vi "runningseperately.vi"() -> ()   [LabVIEW 2019]
uses:
  <vilib>/Utility/file.llb/Read Delimited Spreadsheet (DBL).vi
panel:
  out "Torque Setpoints_graph":dbl(graph)
  in  "Tyre Diameter(m)":sgl=0.78
  in  "file path (dialog if empty)":path=path "C:/Users/arda/Documents/GitHub/labviewtestbench/RPM_setpointfile/wholetest.txt"
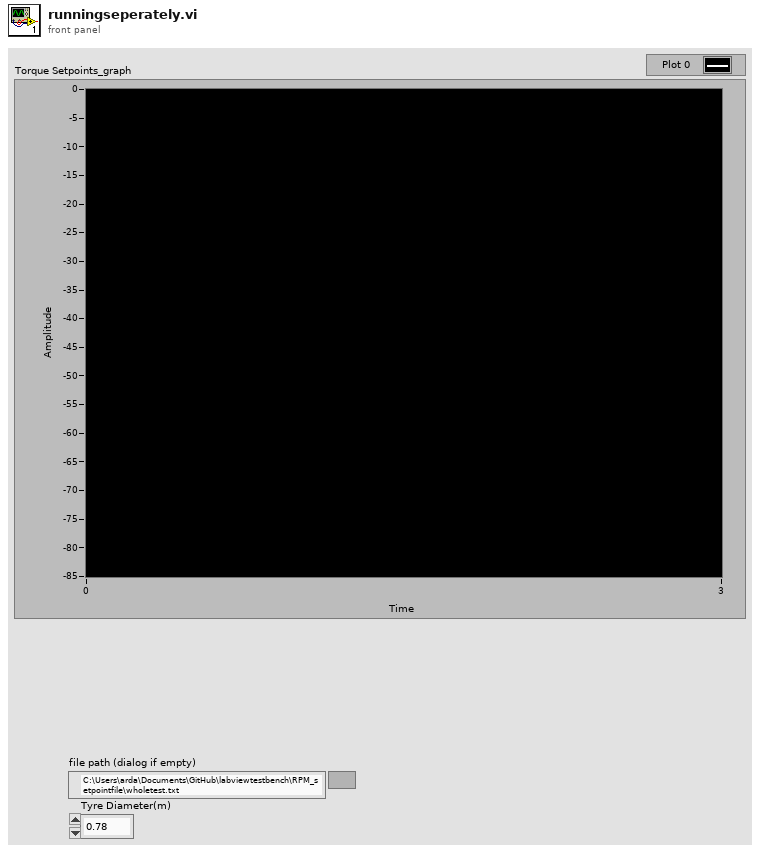
[diagram p1: front panel]
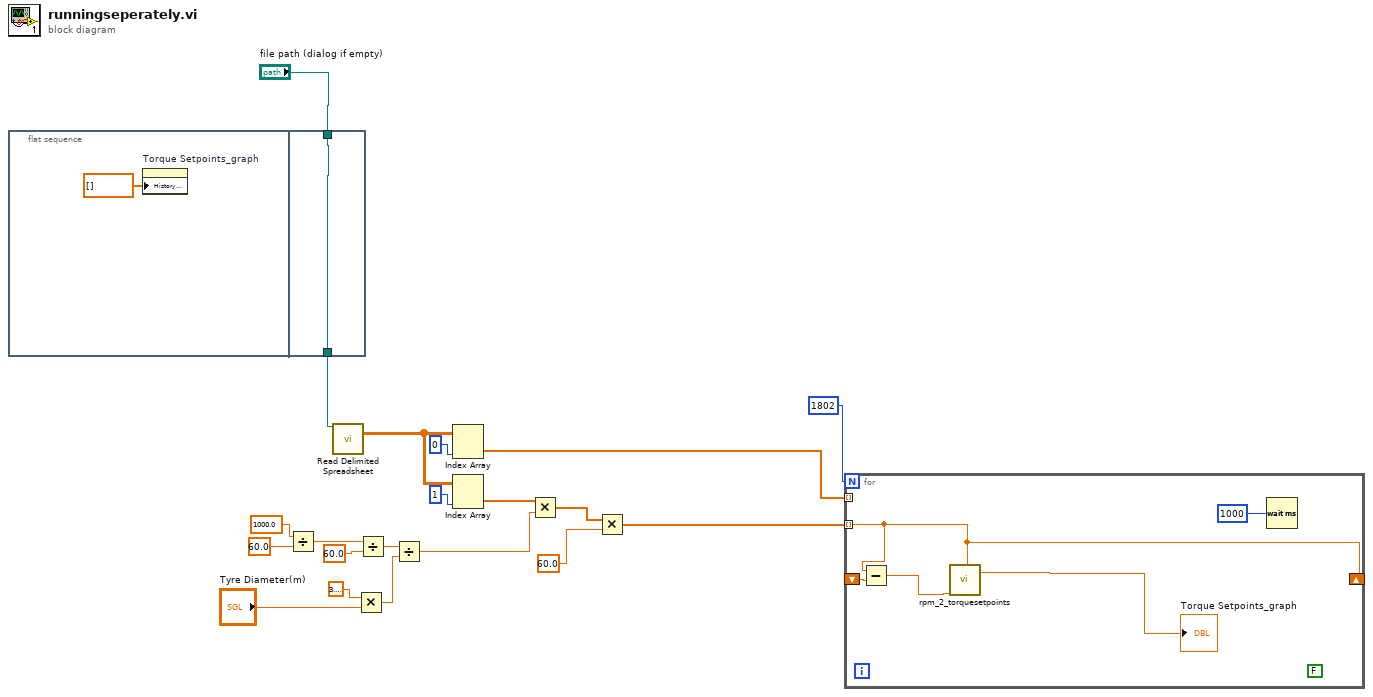
[diagram p0: block diagram]
diagram:
  n1 = flat-sequence {
    tunnel: [w22] -> w2
    tunnel: "file path (dialog if empty)" -> [w22]
    frame #0 {
      n2 = property on="Torque Setpoints_graph" class="WFChart (strict)"("History Data"=dbl[] []) -> ()  [unwired: 2 in, 2 out]
    }
    frame #1 {
    }
  }
  n3 = Divide(x=sgl 1000.0, y=sgl 60.0) -> (x/y=w17:sgl)
  n4 = call-poly <vilib>:"Read Delimited Spreadsheet.vi"("file path (dialog if empty)"=w2) -> ("all rows"=w20:dbl[][])  [unwired: 9 in, 5 out]
  n5 = Multiply(x=sgl 3.1415927, y="Tyre Diameter(m)") -> (x*y=w15:sgl)
  n6 = Divide(x=w17, y=sgl 60.0) -> (x/y=w19:sgl)
  n7 = Divide(x=w19, y=w15) -> (x/y=w9:sgl)
  n8 = Index Array(array=w20, index (col)=0 ("index (row)")) -> (element=w7:dbl[])  [unwired: 1 in]
  n9 = Index Array(array=w20, index (col)=1 ("index (row)")) -> (element=w10:dbl[])  [unwired: 1 in]
  n10 = Multiply(x=w10, y=w9) -> (x*y=w12:dbl[])
  n11 = Multiply(x=w12, y=sgl 60.0) -> (x*y=w8:dbl[])
  n12 = for {
    N: 1802 -> [_]
    tunnel: w8 -> [w25] mode=indexing
    tunnel: w7 -> [_] mode=indexing
    shift-right: [w25] -> _
    shift-left: _ -> [w24]
    (unwired) FALSE
    n13 = Subtract(x=w25, y=w24) -> (x-y=w23:dbl)
    n14 = call "rpm_2_torquesetpoints.vi"("derivative"=w23, "RPM"=w25) -> ("Torque Setpoints"=→"Torque Setpoints_graph":dbl)  [unwired: 10 in, 7 out]
    n15 = Wait (ms)(milliseconds to wait=u32 1000) -> ()  [unwired: 1 out]
  }
